vi "CSDB_Config.set boolean values.vi"(2 "Type":string, 3 "AttributeName":string, 10 "Values in":string[](array[string]), 12 "InstanceNames in":string[](array[string])) -> (16 "Values out":string[](array[string]))   [LabVIEW 2014, in "CSDB_Config.lvlib"]
doc: "Sets a boolean value of an object"
uses:
  CSDB_Config.lvlib
panel:
  in  "cancel":bool
  in  "done":bool
  in  "Table":i32[](listbox)
  in  "set  FALSE":bool
  in  "set TRUE":bool
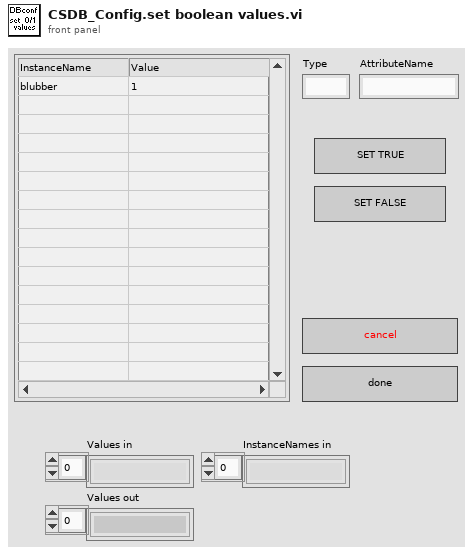
[diagram p1: front panel]
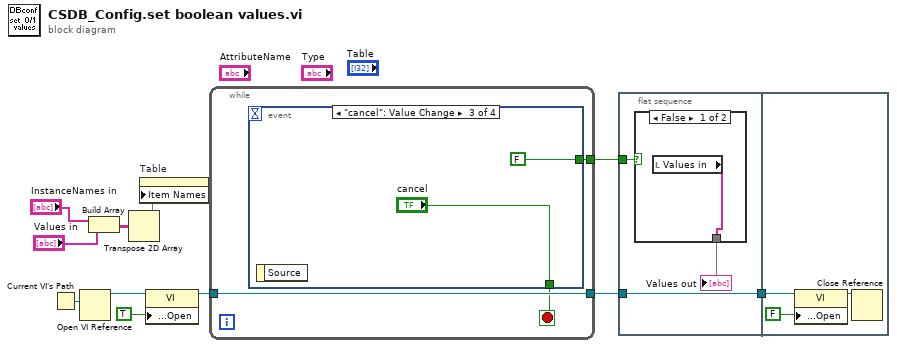
[diagram p0: block diagram]
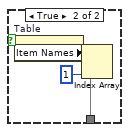
[diagram p2: hidden frame]
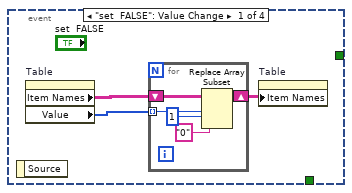
[diagram p3: hidden frame]
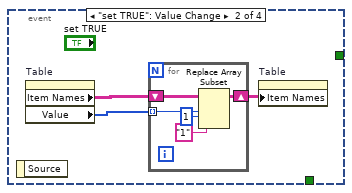
[diagram p4: hidden frame]
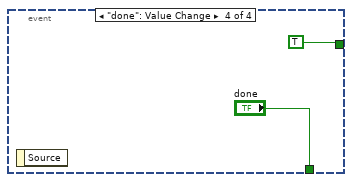
[diagram p5: hidden frame]
diagram:
  n1 = Current VI's Path() -> (path=w11:path)
  n2 = Open VI Reference(vi path=w11) -> (vi reference=w10:refnum<vi>)  [unwired: 5 in, 1 out]
  n3 = Build Array("InstanceNames in", "Values in") -> (w5:string[][])
  n4 = Transpose 2D Array(2D array=w5) -> (transposed array=w4:string[][])
  n5 = property on="Table" class="MCListbox (strict)"("Item Names"=w4) -> ()  [unwired: 2 in, 2 out]
  n6 = property class="VI"(reference=w10, "Front Panel Window:Open"=TRUE) -> (reference out=w8:refnum<vi>)  [unwired: 1 in, 1 out]
  n7 = while {
    tunnel: [w14] -> w3
    tunnel: w8 -> [w14]
    tunnel: [w12] -> w1
    stop <- w13 stop-if-true
    n8 = event shown="[2] \"cancel\": Value Change" {
      selector: _ -> [_ _ _ _]
      dyn-events: _ -> [_ _ _ _]
      timeout: _ -> [_ _ _ _]
      tunnel: [_ _ "cancel" "done"] -> w13
      tunnel: [_ _ FALSE TRUE] -> w12
      event "set  FALSE": Value Change {
        n9 = event-data() -> ()  [unwired: 1 in, 1 out]
        n10 = property on="Table" class="MCListbox (strict)"() -> ("Item Names"=w17:string[][], "Value"=w16:i32[])  [unwired: 2 in, 2 out]
        n11 = for {
          tunnel: w16 -> [w21] mode=indexing
          shift-right: [w18] -> w15
          shift-left: w17 -> [w22]
          n12 = Replace Array Subset(array=w22, new element="0" ("new element/subarray"), index (row)=w21, index (col)=1 ("disabled index (col)")) -> (w18:string[][])
        }
        n13 = property on="Table" class="MCListbox (strict)"("Item Names"=w15) -> ()  [unwired: 2 in, 2 out]
      }
      event "set TRUE": Value Change {
        n14 = event-data() -> ()  [unwired: 1 in, 1 out]
        n15 = property on="Table" class="MCListbox (strict)"() -> ("Item Names"=w25:string[][], "Value"=w24:i32[])  [unwired: 2 in, 2 out]
        n16 = for {
          tunnel: w24 -> [w29] mode=indexing
          shift-right: [w26] -> w23
          shift-left: w25 -> [w30]
          n17 = Replace Array Subset(array=w30, new element="1" ("new element/subarray"), index (row)=w29, index (col)=1 ("disabled index (col)")) -> (w26:string[][])
        }
        n18 = property on="Table" class="MCListbox (strict)"("Item Names"=w23) -> ()  [unwired: 2 in, 2 out]
      }
      event "cancel": Value Change {
        n19 = event-data() -> ()  [unwired: 1 in, 1 out]
      }
      event "done": Value Change {
        n20 = event-data() -> ()  [unwired: 1 in, 1 out]
      }
    }
  }
  n21 = flat-sequence {
    tunnel: w3 -> [w37]
    tunnel: [w37] -> w2
    tunnel: w1 -> [w35]
    tunnel: w2 -> [w42]
    frame #0 {
      n22 = case shown="False" w35 {
        tunnel: [w38 w39] -> w36
        frame False {
          n23 = local read "Values in"() -> (w38:string[])
        }
        frame True {
          n24 = property on="Table" class="MCListbox (strict)"() -> ("Item Names"=w41:string[][])  [unwired: 2 in, 2 out]
          n25 = Index Array(array=w41, index (col)=1 ("disabled index (col)")) -> (element=w39:string[])  [unwired: 1 in]
        }
      }
      "Values out" <- w36
    }
    frame #1 {
      n26 = property class="VI"(reference=w42, "Front Panel Window:Open"=FALSE) -> (reference out=w44:refnum<vi>)  [unwired: 1 in, 1 out]
      n27 = Close Reference(reference=w44) -> ()  [unwired: 1 in, 1 out]
    }
  }
